vi "FTW-ActorExtended-LaunchChildActor-Path.vi"(0 "FTW Actor Connector Type":refnum<class "FTW-ActorExtended.lvclass">, 5 "Configuration":string="{\n  \"Identity\": \"ActorName\",\n  \"DebugEnableInboxLogging\": false,\n  \"DebugEnableJobLogging\": false,\n  \"InboxAddress\": \"inproc://*\",\n  \"DebugShowPanel\": false\n}", 7 "Actor VI Path":path, 9 "Timeout":i32=-2 format="%dmsec", 11 "error in":errorcluster) -> (4 "FTW-ActorExtended.lvclass":refnum<class "FTW-ActorExtended.lvclass">, 6 "Initialized Response":string, 8 "Instance Inbox Address":string, 10 "Identity":string, 15 "error out":errorcluster)   [LabVIEW 2015, in "FTW-ActorExtended.lvclass"]
doc: "This is the spawn new actor that was used for a while. It lacks the minimum strict inputs required to launch an actor."
uses:
  FTW-ActorExtended.lvclass
  Connector/FTW-ActorConnector.lvclass
  JSON/core/FTW-JSON-Core-EncodingFlags.vi
  JSON/FTW-JSON-Parse.vi
  Reflection/FTW-Reflection-Type.vi
  CodeGen/JSON Deserialize/FTW-JSON-Core-GetFlattenedValue.vi
  CodeGen/JSON Deserialize/FTW-JSON-Deserialize.xnode
panel:
  # "Inputs"
  # "Outputs"
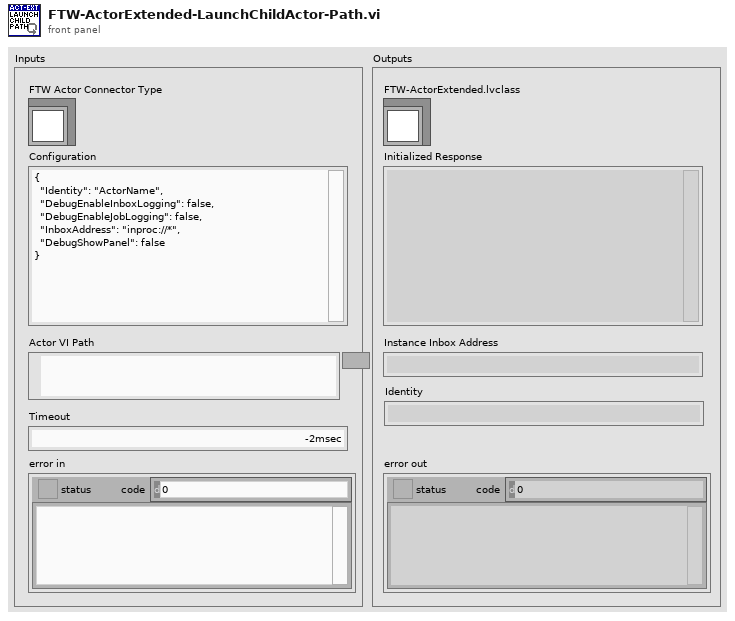
[diagram p1: front panel]
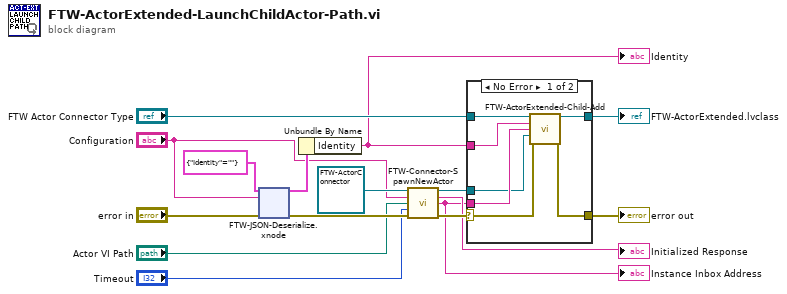
[diagram p0: block diagram]
diagram:
  n1 = xnode "FTW-JSON-Deserialize.xnode"("Type and Defaults"=cluster{"Identity":string} {"Identity"=""}, "JSON String"="Configuration", "error in"="error in") -> ("Values"=w15:cluster{"Identity":string}, "error out"=w13:errorcluster)
  n2 = Unbundle By Name(w15) -> ("Identity"=w2:string)
  "Identity" <- w2
  n3 = call "FTW-Connector-SpawnNewActor.vi"("FTW Actor Connector Type"=refnum<class "FTW-ActorConnector.lvclass"> refnum, "Configuration"="Configuration", "Actor VI Filepath"="Actor VI Path", "Timeout"="Timeout", "error in"=w13) -> ("FTW Actor Connector"=w11:refnum<class "FTW-ActorConnector.lvclass">, "Initialized Response"=→"Initialized Response":string, "Instance Inbox Address"=w5:string, "error out"=w12:errorcluster)  [unwired: 7 in]
  "Instance Inbox Address" <- w5
  n4 = case shown="No Error" w12 {
    selector: w12 -> [w23 w24]
    tunnel: "FTW Actor Connector Type" -> [w21 w25]
    tunnel: [w20 w25] -> w7
    tunnel: [w22 w24] -> w4
    tunnel: w2 -> [w19 _]
    tunnel: w5 -> [w18 _]
    tunnel: w11 -> [w17 _]
    frame No Error {
      n5 = call "FTW-ActorExtended-Child-Add.vi"("FTW-ActorExtended In"=w21, "Identity"=w19, "Inbox Address"=w18, "Connection"=w17, "error in"=w23) -> ("FTW-ActorExtended Out"=w20:refnum<class "FTW-ActorExtended.lvclass">, "error out"=w22:errorcluster)  [unwired: 9 in]
    }
    frame Error {
    }
  }
  "error out" <- w4
  "FTW-ActorExtended.lvclass" <- w7
